vi "曲线查看.vi"(8 "曲线名":string[](array[string]), 11 "曲线数据":sgl[][](array[numeric])) -> (3 "前面板窗口:打开":bool)   [LabVIEW 2020]
panel:
  out "全部曲线":sgl[][](graph)
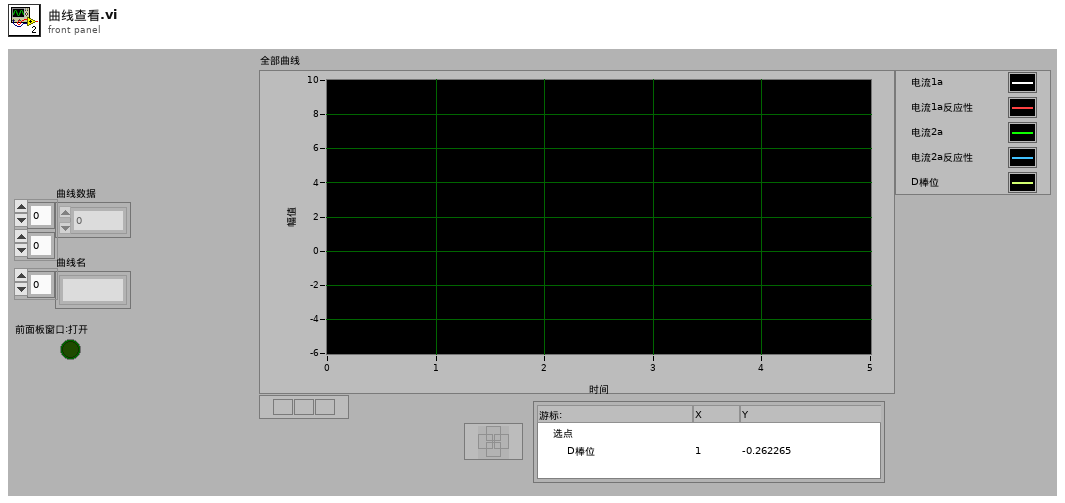
[diagram p1: front panel]
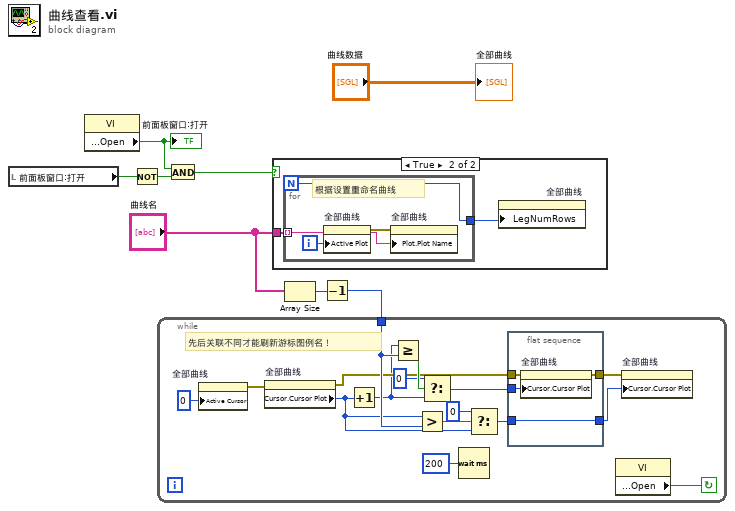
[diagram p0: block diagram]
diagram:
  n1 = local read "前面板窗口:打开"() -> (w4:bool)
  n2 = property class="VI"() -> ("Front Panel.Open"=w2:bool)  [unwired: 2 in, 2 out]
  "前面板窗口:打开" <- w2
  n3 = Not(x=w4) -> (.not. x?=w3:bool)
  n4 = And(x=w2, y=w3) -> (x .and. y?=w5:bool)
  n5 = case shown="True" w5 {
    tunnel: "曲线名" -> [_ w9]
    frame False {
    }
    frame True {
      n6 = for {
        N -> [w11]
        tunnel: w9 -> [w13] mode=indexing
        tunnel: [w11] -> w10
        i -> [w14]
        # "根据设置重命名曲线"
        n7 = property on="全部曲线" class="WFGraph (strict)"("Active Plot"=w14) -> (error out=w12:errorcluster)  [unwired: 2 in, 1 out]
        n8 = property on="全部曲线" class="WFGraph (strict)"(error in=w12, "Plot.Plot Name"=w13) -> ()  [unwired: 1 in, 2 out]
      }
      n9 = property on="全部曲线" class="WFGraph (strict)"("LegNumRows"=w10) -> ()  [unwired: 2 in, 2 out]
    }
  }
  n10 = Array Size(array="曲线名") -> (size(s)=w6:i32)
  n11 = Decrement(x=w6) -> (x-1=w8:i32)
  n12 = while {
    tunnel: w8 -> [w30]
    stop <- w16 continue-if-true
    # "先后关联不同才能刷新游标图例名！"
    n13 = property on="全部曲线" class="WFGraph (strict)"("Active Cursor"=u32 0 ("活动游标")) -> (error out=w29:errorcluster)  [unwired: 2 in, 1 out]
    n14 = property on="全部曲线" class="WFGraph (strict)"(error in=w29) -> (error out=w26:errorcluster, "Cursor.Cursor Plot"=w21:i32)  [unwired: 1 in, 1 out]
    n15 = Increment(x=w21) -> (x+1=w20:i32)
    n16 = Greater Or Equal?(x=w20, y=w30) -> (x >= y?=w28:bool)
    n17 = Greater?(x=w21, y=w30) -> (0:w23:bool)
    n18 = Select(t=0, s=w28, f=w20) -> (s? t:f=w25:i32)
    n19 = Wait (ms)(milliseconds to wait=u32 200 ("等待时间（毫秒）")) -> ()  [unwired: 1 out]
    n20 = Select(t=0, s=w23, f=w21) -> (s? t:f=w19:i32)
    n21 = flat-sequence {
      tunnel: [w34] -> w27
      tunnel: w26 -> [w33]
      tunnel: w25 -> [w32]
      tunnel: w19 -> [w31]
      tunnel: [w31] -> w18
      frame #0 {
        n22 = property on="全部曲线" class="WFGraph (strict)"(error in=w33, "Cursor.Cursor Plot"=w32) -> (error out=w34:errorcluster)  [unwired: 1 in, 1 out]
      }
    }
    n23 = property class="VI"() -> ("Front Panel.Open"=w16:bool)  [unwired: 2 in, 2 out]
    n24 = property on="全部曲线" class="WFGraph (strict)"(error in=w27, "Cursor.Cursor Plot"=w18) -> ()  [unwired: 1 in, 2 out]
  }
  "全部曲线" <- "曲线数据"
